vi "8601 UTC Date-Time String.vi"(0 "Time Part (HH:MM:SS)":u16(ring) items=["HH:MM:SS", "HH:MM", "HH", ""], 1 "Date Part (YYYY-mm-dd)":u16(ring) items=["YYYY-mm-dd", "YYYY-ww-d", "YYYY-ddd", "YYYY-ww", "YYYY-mm", "YY-mm-dd", "YY-ww-d", "YY-ddd", "YY-ww", "YY-mm"], 2 "Zulu? (F)":bool, 7 "time stamp (Current Time)":timestamp format="%<%X\n%x>T", 11 "error in (no error)":errorcluster, 12 "Include TZ? (T)":bool=TRUE, 13 "Basic? (F)":bool) -> (4 "8601 Date/Time String":string, 8 "time stamp out":timestamp=timestamp(3313630800 s since 1904-01-01) format="%<%X\n%a %x>T", 15 "error out":errorcluster)   [LabVIEW 2020, in "XML Report.lvclass"]
doc: "Returns an extended ISO 8601 UTC Combined Date/Time string. If time stamp is not specified, the current date/time is used and returned in time stamp out.\n\nSet<B> Basic?</B> to <B>TRUE</B> if you want a compact Date/Time string (no date and time separators).\n \nFor info regarding 8601 string formatting, see: http://en.wikipedia.org/wiki/ISO_8601"
uses:
  XML Report.lvclass
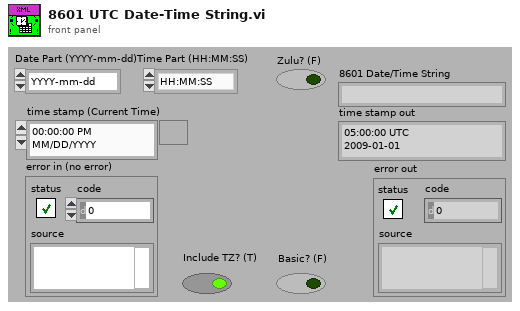
[diagram p1: front panel]
types:
  T1 = typedef "LVDateTimeRec.ctl" = cluster{"fractional second":dbl, "second":i32, "minute":i32, "hour":i32, "day of month":i32, "month":i32, "year":i32, "day of week":i32, "day of year":i32, "DST":i32}
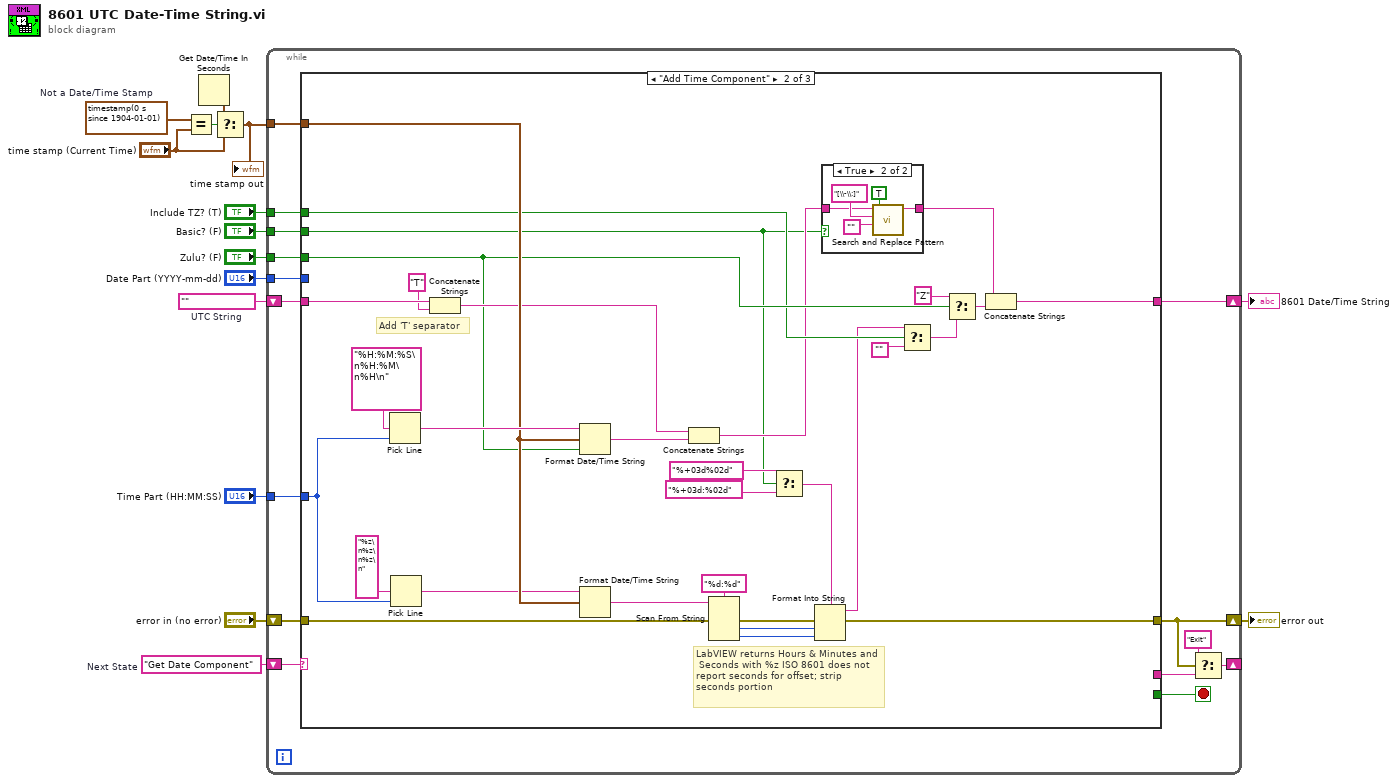
[diagram p0: block diagram]
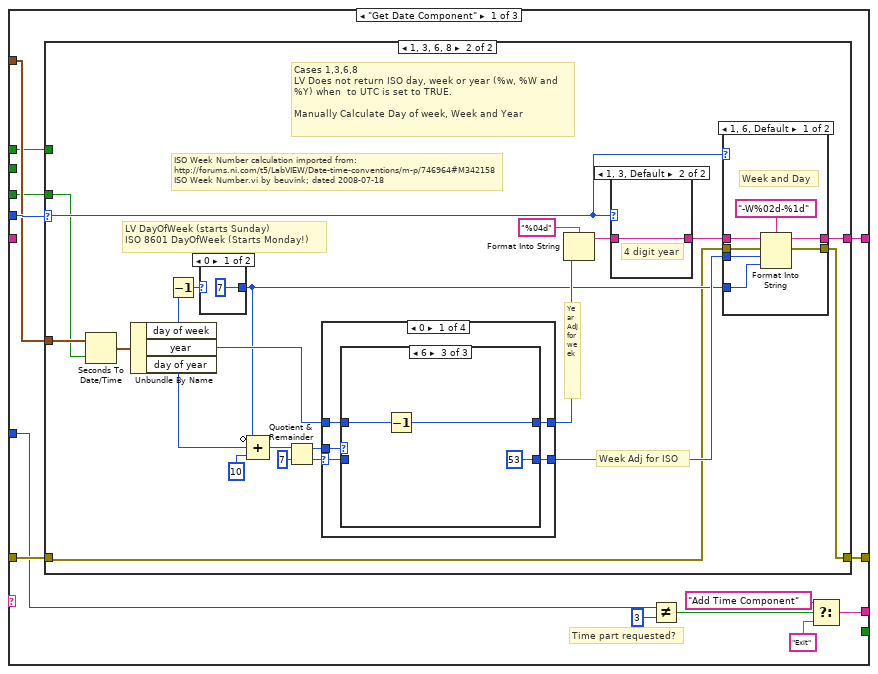
[diagram p2: hidden frame]
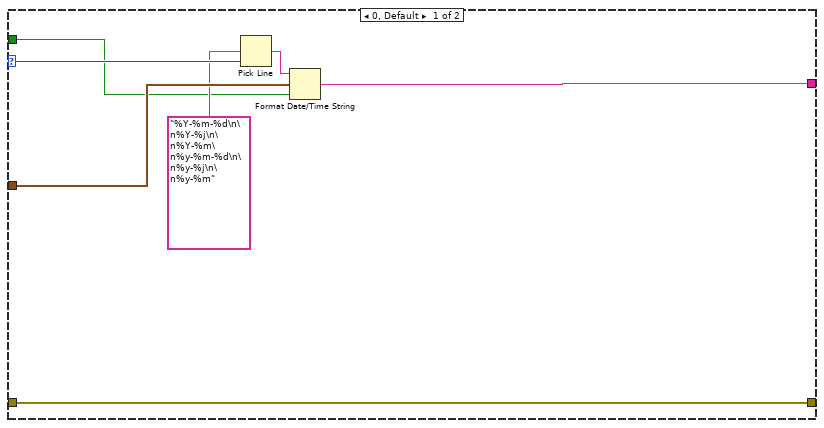
[diagram p3: hidden frame]
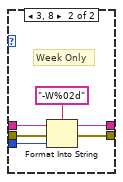
[diagram p4: hidden frame]
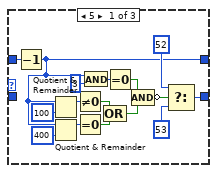
[diagram p5: hidden frame]
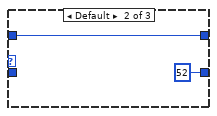
[diagram p6: hidden frame]
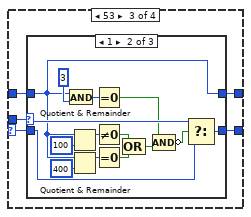
[diagram p8: hidden frame]
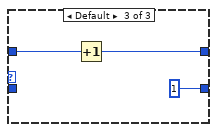
[diagram p10: hidden frame]
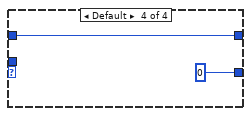
[diagram p11: hidden frame]
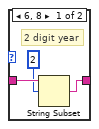
[diagram p13: hidden frame]
diagram:
  w10 = "Get Date Component"  # Next State
  w11 = ""  # UTC String
  w12 = timestamp(0 s since 1904-01-01)  # Not a Date/Time Stamp
  n1 = Equal?(x=w12, y="time stamp (Current Time)") -> (x = y?=w14:bool)
  n2 = Get Date/Time In Seconds() -> (seconds since 1Jan1904=w15:timestamp)
  n3 = Select(t=w15, s=w14, f="time stamp (Current Time)") -> (s? t:f=w8:timestamp)
  "time stamp out" <- w8
  n4 = while {
    shift-right: [w29] -> w1
    shift-left: w11 -> [w28]
    shift-right: [w16] -> _
    shift-left: w10 -> [w30]
    tunnel: "Date Part (YYYY-mm-dd)" -> [w27]
    tunnel: w8 -> [w26]
    tunnel: "Zulu? (F)" -> [w25]
    tunnel: "Include TZ? (T)" -> [w24]
    shift-right: [w19] -> w4
    shift-left: "error in (no error)" -> [w23]
    tunnel: "Time Part (HH:MM:SS)" -> [w22]
    tunnel: "Basic? (F)" -> [w20]
    stop <- w21 stop-if-true
    n5 = case shown="\"Add Time Component\"" w30 {
      tunnel: [w43 "Exit" "Exit"] -> w17
      tunnel: [w36 w147 w188] -> w29
      tunnel: w28 -> [_ w175 w188]
      tunnel: w27 -> [w38 _ _]
      tunnel: w26 -> [w37 w165 _]
      tunnel: w25 -> [w31 w160 _]
      tunnel: w24 -> [w33 w154 _]
      tunnel: w23 -> [w34 w178 w187]
      tunnel: [w35 w177 w187] -> w19
      tunnel: w22 -> [w32 w172 _]
      tunnel: [_ _ TRUE] -> w21
      tunnel: w20 -> [_ w150 _]
      frame "Get Date Component" {
        # "Time part requested?"
        n6 = case shown="1, 3, 6, 8" w38 {
          selector: w38 -> [w50 w52]
          tunnel: w37 -> [w49 w55]
          tunnel: [w47 w56] -> w36
          tunnel: [w46 w54] -> w35
          tunnel: w34 -> [w46 w53]
          tunnel: w33 -> [_ _]
          tunnel: w31 -> [w44 w51]
          frame 0, Default {
            n7 = Pick Line(multi-line string="%Y-%m-%d\n\n%Y-%j\n\n%Y-%m\n%y-%m-%d\n\n%y-%j\n\n%y-%m", line index=w50) -> (output string=w48:string)  [unwired: 1 out]
            n8 = Format Date/Time String(time format string (%c)=w48, seconds (now)=w49, UTC format=w44) -> (date/time string=w47:string)
          }
          frame 1, 3, 6, 8 {
            # "ISO Week Number calculation imported from:\nhttp://forums.ni.com/t5/LabVIEW/Date-time-conventions/m-p/746964#M342158\nISO Week Number.vi by beuvink; dated 2008-07-18"
            # "Cases 1,3,6,8\nLV Does not return ISO day, week or year (%w, %W and %Y) when  to UTC is set to TRUE.\n\nManually Calculate Day of week, Week and Year"
            # "Week Adj for ISO"
            # "Year Adj for week"
            # "LV DayOfWeek (starts Sunday)\nISO 8601 DayOfWeek (Starts Monday!)"
            n9 = Seconds To Date/Time(time stamp (now)=w55, to UTC (F)=w51) -> (date time rec=w66:T1)
            n10 = Unbundle By Name(w66) -> ("day of week"=w71:i32, "year"=w63:i32, "day of year"=w72:i32)
            n11 = Decrement(x=w71) -> (x-1=w70:i32)
            n12 = case shown="0" w70 {
              selector: w70 -> [_ w142]
              tunnel: [7 ("day of week") w142] -> w57
              frame 0 {
              }
              frame Default {
              }
            }
            n13 = Compound Arithmetic op=ADD(invert w57, w72, 10 ("Input")) -> (w68:i32)
            n14 = Quotient & Remainder(x=w68, y=7) -> (x-y*floor(x/y)=w64:i32, floor(x/y)=w65:i32)
            n15 = case shown="0" w65 {
              selector: w65 -> [w90 w113 w116 _]
              tunnel: [w88 w113 w117 0] -> w58
              tunnel: w64 -> [w89 _ w118 _]
              tunnel: w63 -> [w87 w112 w115 w139]
              tunnel: [w86 w112 w114 w139] -> w61
              frame 0 {
                n16 = case shown="6" w89 {
                  tunnel: [w106 52 ("t") 53 ("t")] -> w88
                  tunnel: w90 -> [_ _ _]
                  tunnel: w87 -> [w92 w107 w110]
                  tunnel: [w91 w107 w109] -> w86
                  frame 5 {
                    n17 = Decrement(x=w92) -> (x-1=w91:i32)
                    n18 = Quotient & Remainder(x=w91, y=100) -> (x-y*floor(x/y)=w103:i32)  [unwired: 1 out]
                    n19 = Quotient & Remainder(x=w91, y=400) -> (x-y*floor(x/y)=w104:i32)  [unwired: 1 out]
                    n20 = Not Equal To 0?(x=w103) -> (x != 0?=w98:bool)
                    n21 = Equal To 0?(x=w104) -> (x = 0?=w97:bool)
                    n22 = And(x=w91, y=3) -> (x .and. y?=w102:i32)
                    n23 = Compound Arithmetic op=OR(w98, w97) -> (w96:bool)
                    n24 = Equal To 0?(x=w102) -> (x = 0?=w105:bool)
                    n25 = Compound Arithmetic op=AND(w105, w96) -> (invert w99:bool)
                    n26 = Select(t=52, s=w99, f=53 ("t")) -> (s? t:f=w106:i32)
                  }
                  frame Default {
                  }
                  frame 6 {
                    n27 = Decrement(x=w110) -> (x-1=w109:i32)
                  }
                }
              }
              frame 1..52 {
              }
              frame 53 {
                n28 = case shown="1" w118 {
                  selector: w118 -> [_ w134 _]
                  tunnel: [w120 w135 1] -> w117
                  tunnel: w116 -> [w120 w133 _]
                  tunnel: w115 -> [w119 w121 w137]
                  tunnel: [w119 w121 w136] -> w114
                  frame 0 {
                  }
                  frame 1 {
                    n29 = And(x=w121, y=3) -> (x .and. y?=w129:i32)
                    n30 = Quotient & Remainder(x=w121, y=100) -> (x-y*floor(x/y)=w130:i32)  [unwired: 1 out]
                    n31 = Quotient & Remainder(x=w121, y=400) -> (x-y*floor(x/y)=w131:i32)  [unwired: 1 out]
                    n32 = Equal To 0?(x=w129) -> (x = 0?=w132:bool)
                    n33 = Not Equal To 0?(x=w130) -> (x != 0?=w124:bool)
                    n34 = Equal To 0?(x=w131) -> (x = 0?=w123:bool)
                    n35 = Compound Arithmetic op=OR(w124, w123) -> (w122:bool)
                    n36 = Compound Arithmetic op=AND(w132, w122) -> (invert w125:bool)
                    n37 = Select(t=w134, s=w125, f=w133) -> (s? t:f=w135:i32)
                  }
                  frame Default {
                    n38 = Increment(x=w137) -> (x+1=w136:i32)
                  }
                }
              }
              frame Default {
              }
            }
            n39 = Format Into String(format string="%04d", w61) -> (resulting string=w60:string)  [unwired: 2 in, 1 out]
            n40 = case shown="1, 3, Default" w52 {
              tunnel: w60 -> [w145 w146]
              tunnel: [w143 w146] -> w59
              frame 6, 8 {
                # "2 digit year"
                n41 = String Subset(string=w145, offset (0)=2) -> (substring=w143:string)  [unwired: 1 out]
              }
              frame 1, 3, Default {
                # "4 digit year"
              }
            }
            n42 = case shown="1, 6, Default" w52 {
              tunnel: w59 -> [w79 w85]
              tunnel: w58 -> [w77 w83]
              tunnel: w57 -> [w76 _]
              tunnel: [w75 w82] -> w56
              tunnel: [w74 w81] -> w54
              tunnel: w53 -> [w73 w80]
              frame 1, 6, Default {
                # "Week and Day"
                n43 = Format Into String(format string="-W%02d-%1d", initial string=w79, error in=w73, w77, w76) -> (resulting string=w75:string, error out=w74:errorcluster)
              }
              frame 3, 8 {
                # "Week Only"
                n44 = Format Into String(format string="-W%02d", initial string=w85, error in=w80, w83) -> (resulting string=w82:string, error out=w81:errorcluster)
              }
            }
          }
        }
        n45 = Not Equal?(x=w32, y=u16 3) -> (x != y?=w40:bool)
        n46 = Select(t="Add Time Component", s=w40, f="Exit") -> (s? t:f=w43:string)
      }
      frame "Add Time Component" {
        # "Add 'T' separator"
        # "LabVIEW returns Hours & Minutes and\n Seconds with %z ISO 8601 does not report seconds for offset; strip seconds portion"
        n47 = Pick Line(multi-line string="%H:%M:%S\n%H:%M\n%H\n", line index=w172) -> (output string=w166:string)  [unwired: 1 out]
        n48 = Pick Line(multi-line string="%z\n%z\n%z\n", line index=w172) -> (output string=w164:string)  [unwired: 1 out]
        n49 = Concatenate Strings(w175, "T" ("string")) -> (w162:string)
        n50 = Format Date/Time String(time format string (%c)=w166, seconds (now)=w165, UTC format=w160) -> (date/time string=w161:string)
        n51 = Format Date/Time String(time format string (%c)=w164, seconds (now)=w165) -> (date/time string=w163:string)  [unwired: 1 out]
        n52 = Concatenate Strings(w162, w161) -> (w151:string)
        n53 = Scan From String(format string="%d:%d", input string=w163, error in=w178) -> (error out=w167:errorcluster, output 1=w169:i32, output 2=w168:i32)  [unwired: 1 in, 4 out]
        n54 = Select(t="%+03d%02d" ("format string"), s=w150, f="%+03d:%02d" ("format string")) -> (s? t:f=w157:string)
        n55 = Format Into String(format string=w157, error in=w167, w169, w168) -> (resulting string=w153:string, error out=w177:errorcluster)  [unwired: 1 in]
        n56 = case shown="True" w150 {
          tunnel: w151 -> [w179 w182]
          tunnel: [w179 w180] -> w149
          frame False {
          }
          frame True {
            n57 = call <vilib>:"Search and Replace Pattern.vi"("string"=w182, "regular expression (\"\")"="[\\-\\:]" ("search string"), "replace string (\"\")"="", "replace all? (F)"=TRUE) -> ("result string"=w180:string)  [unwired: 2 out]
          }
        }
        n58 = Select(t=w153, s=w154, f="") -> (s? t:f=w148:string)
        n59 = Select(t="Z", s=w160, f=w148) -> (s? t:f=w156:string)
        n60 = Concatenate Strings(w149, w156) -> (w147:string)
      }
      frame "Exit", Default {
      }
    }
    n61 = Select(t="Exit", s=w19, f=w17) -> (s? t:f=w16:string)
  }
  "8601 Date/Time String" <- w1
  "error out" <- w4
